vi "MCP Reset.vi"(8 "error in (no error)":errorcluster) -> (0 "error out":errorcluster)   [LabVIEW 2020]
uses:
  bbf8e5b3-6ca3-468b-b806-0045224ef793.vi
  MCP2221A LabVIEW library/Microchip MCP2221A_64bit/VIs/Private/mcp2221_dll_um_x64.dll
panel:
  out "noOfDevs out":u32=1
  out "handle out":u64
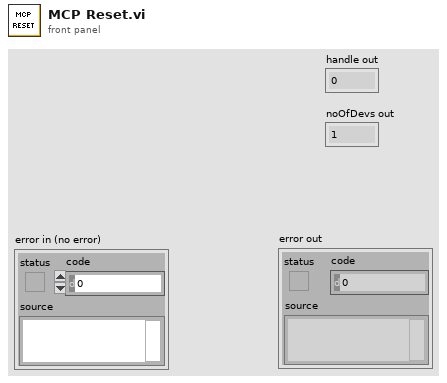
[diagram p1: front panel]
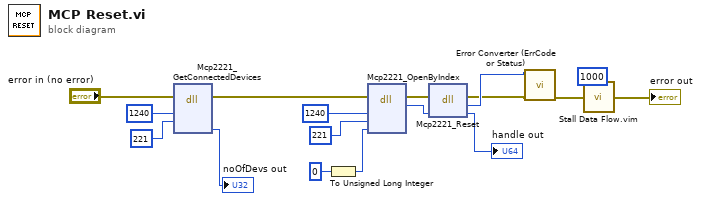
[diagram p0: block diagram]
diagram:
  n1 = dll-call lib="C:/Users/tuguialexand/Desktop/Licenta/MCP2221A LabVIEW library/Microchip MCP2221A_64bit/VIs/Private/mcp2221_dll_um_x64.dll" fn="Mcp2221_GetConnectedDevices"(error in="error in (no error)", "vid"=u32 1240, "pid"=u32 221) -> (error out=w3:errorcluster, "noOfDevs"=→"noOfDevs out":u32)  [unwired: 6 in, 1 out]
  n2 = To Unsigned Long Integer(number=0 ("index")) -> (unsigned 32bit integer=w6:u32)
  n3 = dll-call lib="C:/Users/tuguialexand/Desktop/Licenta/MCP2221A LabVIEW library/Microchip MCP2221A_64bit/VIs/Private/mcp2221_dll_um_x64.dll" fn="Mcp2221_OpenByIndex"(error in=w3, "VID"=u32 1240, "PID"=u32 221, "index"=w6) -> (error out=w2:errorcluster, "return type"=w1:u64)  [unwired: 5 in, 1 out]
  n4 = dll-call lib="C:/Users/tuguialexand/Desktop/Licenta/MCP2221A LabVIEW library/Microchip MCP2221A_64bit/VIs/Private/mcp2221_dll_um_x64.dll" fn="Mcp2221_Reset"(error in=w2, "handle"=w1) -> (error out=w15:errorcluster, "return type"=w16:i32, "handle"=→"handle out":u64)  [unwired: 2 in, 1 out]
  n5 = call "Error Converter (ErrCode or Status).vi"("error code"=w16, "error in (no error)"=w15) -> ("error out"=w14:errorcluster)  [unwired: 13 in]
  n6 = call "Stall Data Flow.vim"("value in"=w14, "milliseconds to wait"=u32 1000) -> ("value out"=→"error out":errorcluster)  [unwired: 1 out]
